vi "loadTF_resample.vi"(9 "desired freqs":dbl[](array[numeric]), 10 "mat file name":string="2021-11-04_TF_Rx_HamburgV2b_G100_Butler_VperM.mat") -> (1 "TF units from loaded file":string, 2 "output TF phase":dbl[](array[numeric]), 3 "output TF mag":dbl[](array[numeric]))   [LabVIEW 2021]
panel:
  out "abs(TF)":cluster{"desired freqs":dbl[], dbl[]}[](graph)
  out "TF_VperM":cdb[](array[numeric])
  out "input freq":dbl[](array[numeric])
  out "input TF_VperM":cdb[](array[numeric])
  out "path for measured TF mat file":path=path "C:/Users/MPI/Documents/GitHub/LabviewGUI/Transfer function load"
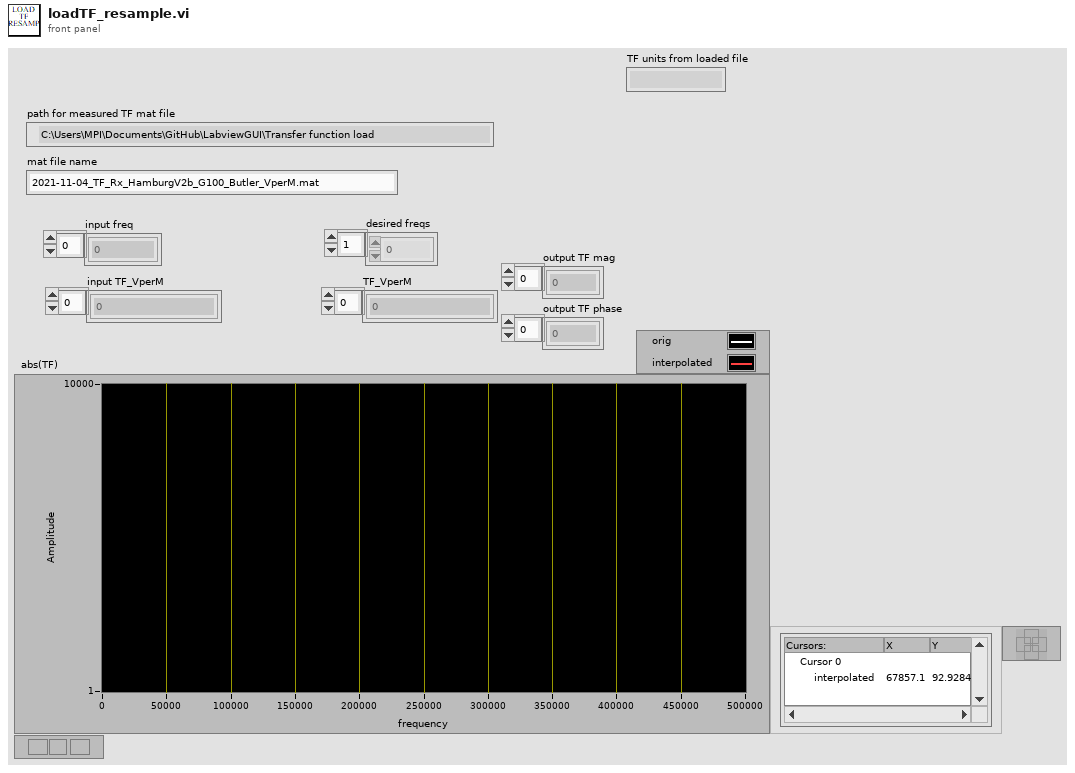
[diagram p1: front panel]
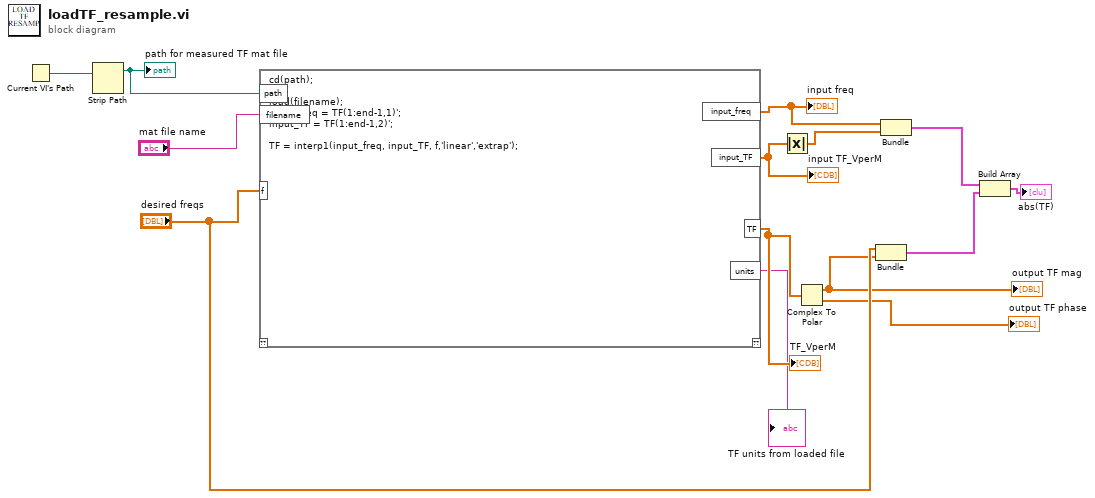
[diagram p0: block diagram]
diagram:
  n1 = Current VI's Path() -> (path=w14:path)
  n2 = Strip Path(path=w14) -> (stripped path=w13:path)  [unwired: 1 out]
  "path for measured TF mat file" <- w13
  n3 = script code="cd(path);\n\nload(filename);\ninput_freq = TF(1:end-1,1)';\ninput_TF = TF(1:end-1,2)';\n\nTF = interp1(input_freq, input_TF, f,'linear','extrap');"("path"=w13, "filename"="mat file name", "f"="desired freqs") -> ("input_freq"=w11:dbl[], "input_TF"=w9:cdb[], "TF"=w4:cdb[], "units"=→"TF units from loaded file":string)  [unwired: 1 in, 1 out]
  "input TF_VperM" <- w9
  "input freq" <- w11
  "TF_VperM" <- w4
  n4 = Absolute Value(x=w9) -> (abs(x)=w8:dbl[])
  n5 = Complex To Polar(r * e^(i*theta)=w4) -> (r=w3:dbl[], theta=→"output TF phase":dbl[])
  "output TF mag" <- w3
  n6 = Bundle("desired freqs"="desired freqs", w3) -> (w7:cluster{"desired freqs":dbl[], dbl[]})  [unwired: 1 in]
  n7 = Bundle(w11, w8) -> (w6:cluster{dbl[], dbl[]})  [unwired: 1 in]
  n8 = Build Array(w6, w7) -> (→"abs(TF)":cluster{"desired freqs":dbl[], dbl[]}[])
